vi "Launch DQMH Tools by menu.vi"(5 "Project":string="Project", 7 "Application Instance":refnum<vi>, 8 "error in":errorcluster, 10 "Module Ref":refnum<vi>, 11 "DQMH Tools":T1) -> (0 "error out":errorcluster)   [LabVIEW 2019, in "Panther Dashboard.lvlib"]
doc: "Launch a DQMH scripting tool by typing one of the following strings in Quick Drop before pressing the Ctrl-Key shortcut for this plugin:\n\nCreate New DQMH Event - ae, new event, add event, create event, \"\" (empty string)\nRename DQMH Event - re, rename event\nRemove DQMH Event - rme, remove\nConvert DQMH Event - ce, convert\nAdd New DQMH Module - am, new mod, add mod, create mod\nRename DQMH Module - rm, rename module\nValidate DQMH Module - vm, validate\nCreate DQMH Module Template - ct, template\nCreate RT Tester - crt, rt\nNew DQMH Unit Test - cut, unit\n\nDefault Shortcut - [E]"
uses:
  Panther Dashboard.lvlib
  DQMH Tools Menu--enum.ctl
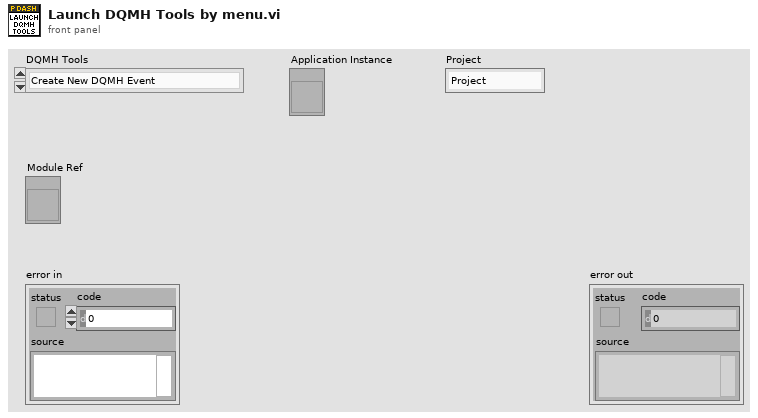
[diagram p1: front panel]
types:
  T1 = typedef "Panther Dashboard.lvlib/DQMH Tools Menu--enum.ctl" = enum16{"Create New DQMH Event", "Remove DQMH Event", "Convert DQMH Event", "Rename DQMH Event", "Add New DQMH Module", "Create RT Tester", "Rename DQMH Module", "Validate DQMH Module", "Create DQMH Module Template", "New DQMH  Unit Test"}
  T2 = enum32{"Invalid", "Standard", "Closed", "Hidden", "Minimized", "Maximized"}
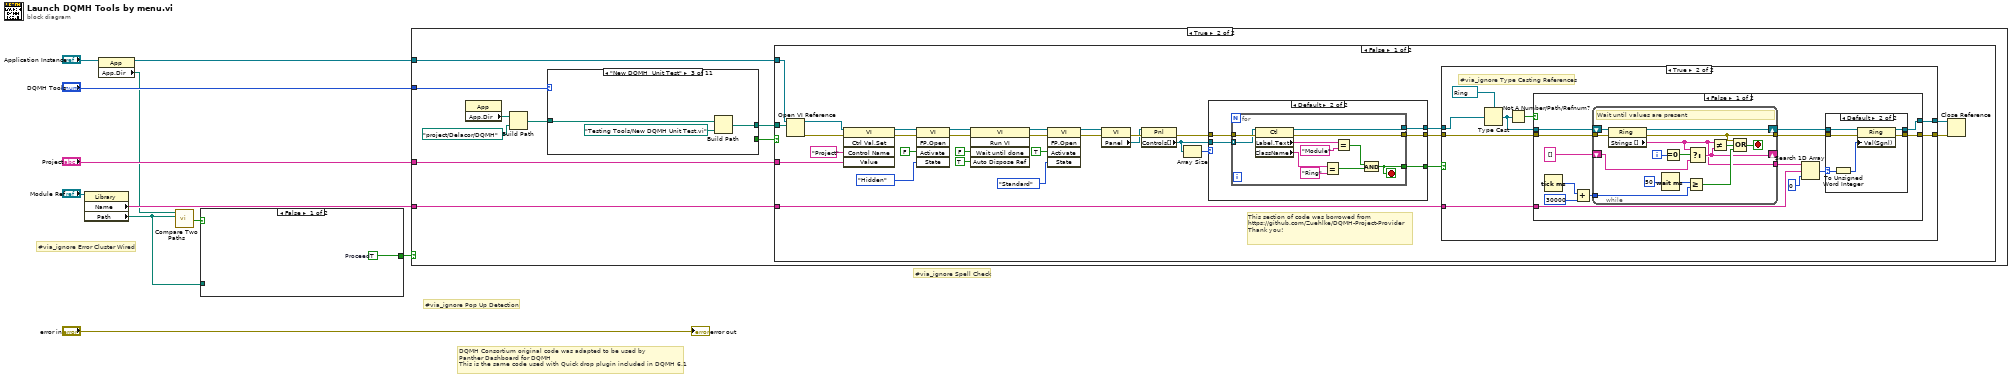
[diagram p0: block diagram]
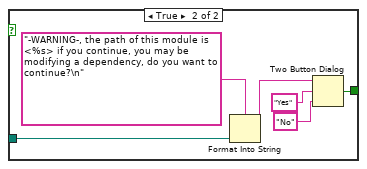
[diagram p2: hidden frame]
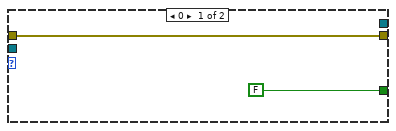
[diagram p4: hidden frame]
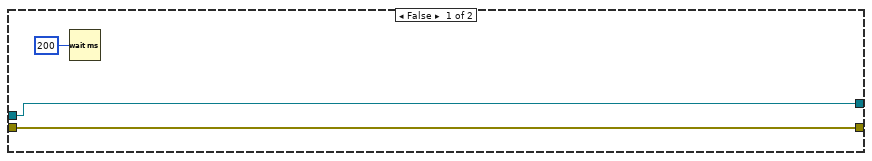
[diagram p5: hidden frame]
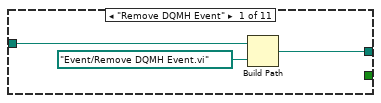
[diagram p9: hidden frame]
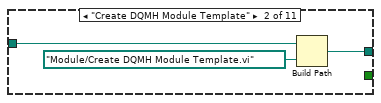
[diagram p10: hidden frame]
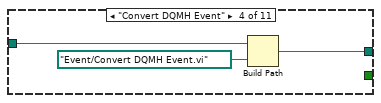
[diagram p11: hidden frame]
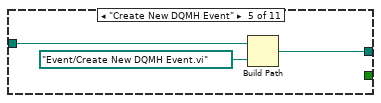
[diagram p12: hidden frame]
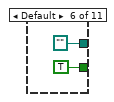
[diagram p13: hidden frame]
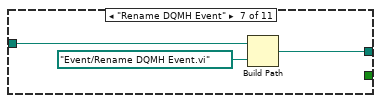
[diagram p14: hidden frame]
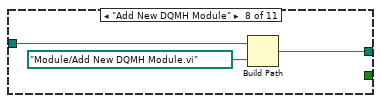
[diagram p15: hidden frame]
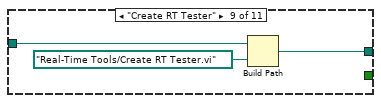
[diagram p16: hidden frame]
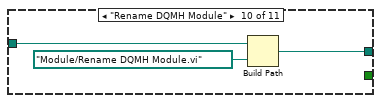
[diagram p17: hidden frame]
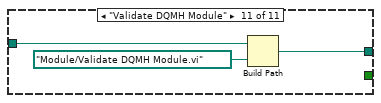
[diagram p18: hidden frame]
diagram:
  # "#via_ignore Error Cluster Wired"
  # "#via_ignore Pop Up Detection"
  # "#via_ignore Spell Check"
  # "DQMH Consortium original code was adapted to be used by \nPanther Dashboard for DQMH\nThis is the same code used with Quick drop plugin included in DQMH 6.1"
  n1 = property class="Library"(reference="Module Ref") -> ("Name"=w8:string, "Path"=w1:path)  [unwired: 1 in, 2 out]
  n2 = property class="App"(reference="Application Instance") -> (reference out=w4:refnum<vi>, "App.Dir"=w3:path)  [unwired: 1 in, 1 out]
  n3 = call <vilib>:"Compare Two Paths.vi"("Path 2"=w1, "Path 1"=w3) -> ("Path 2 Relative to Path 1?"=w2:bool)  [unwired: 6 in, 3 out]
  n4 = case shown="False" w2 {
    tunnel: [w12 w18] -> w6
    tunnel: w1 -> [_ w13]
    frame False {
      w12 = TRUE  # Proceed
    }
    frame True {
      n5 = Format Into String(format string="-WARNING-, the path of this module is <%s> if you continue, you may be modifying a dependency, do you want to continue?\n" ("message"), w13) -> (resulting string=w14:string)  [unwired: 2 in, 1 out]
      n6 = Two Button Dialog(message=w14, 1:"No" ("F button name (\"Cancel\")"), 2:"Yes" ("T button name (\"OK\")")) -> (T button?=w18:bool)
    }
  }
  n7 = case shown="True" w6 {
    tunnel: "DQMH Tools" -> [_ w23]
    tunnel: "Project" -> [_ w21]
    tunnel: w4 -> [_ w20]
    tunnel: w8 -> [_ w19]
    frame False {
    }
    frame True {
      n8 = property class="App"() -> ("App.Dir"=w27:path)  [unwired: 2 in, 2 out]
      n9 = Build Path(base path=w27, name or relative path=path "project/Delacor/DQMH" ("Application:Directory Path")) -> (appended path=w25:path)
      n10 = case shown="\"New DQMH  Unit Test\"" w23 {
        tunnel: w25 -> [w129 w132 w135 w138 w141 _ w146 w149 w152 w155 w158]
        tunnel: [w128 w131 w134 w137 w140 path "" w145 w148 w151 w154 w157] -> w24
        tunnel: [_ _ _ _ _ TRUE _ _ _ _ _] -> w22
        frame "Remove DQMH Event" {
          n11 = Build Path(base path=w129, name or relative path=path "Event/Remove DQMH Event.vi") -> (appended path=w128:path)
        }
        frame "Create DQMH Module Template" {
          n12 = Build Path(base path=w132, name or relative path=path "Module/Create DQMH Module Template.vi") -> (appended path=w131:path)
        }
        frame "New DQMH  Unit Test" {
          n13 = Build Path(base path=w135, name or relative path=path "Testing Tools/New DQMH Unit Test.vi") -> (appended path=w134:path)
        }
        frame "Convert DQMH Event" {
          n14 = Build Path(base path=w138, name or relative path=path "Event/Convert DQMH Event.vi") -> (appended path=w137:path)
        }
        frame "Create New DQMH Event" {
          n15 = Build Path(base path=w141, name or relative path=path "Event/Create New DQMH Event.vi") -> (appended path=w140:path)
        }
        frame Default {
        }
        frame "Rename DQMH Event" {
          n16 = Build Path(base path=w146, name or relative path=path "Event/Rename DQMH Event.vi") -> (appended path=w145:path)
        }
        frame "Add New DQMH Module" {
          n17 = Build Path(base path=w149, name or relative path=path "Module/Add New DQMH Module.vi") -> (appended path=w148:path)
        }
        frame "Create RT Tester" {
          n18 = Build Path(base path=w152, name or relative path=path "Real-Time Tools/Create RT Tester.vi") -> (appended path=w151:path)
        }
        frame "Rename DQMH Module" {
          n19 = Build Path(base path=w155, name or relative path=path "Module/Rename DQMH Module.vi") -> (appended path=w154:path)
        }
        frame "Validate DQMH Module" {
          n20 = Build Path(base path=w158, name or relative path=path "Module/Validate DQMH Module.vi") -> (appended path=w157:path)
        }
      }
      n21 = case shown="False" w22 {
        tunnel: w24 -> [w45 _]
        tunnel: w21 -> [w37 _]
        tunnel: w20 -> [w36 _]
        tunnel: w19 -> [w28 _]
        frame False {
          # "This section of code was borrowed from\nhttps://github.com/Zuehlke/DQMH-Project-Provider\nThank you!"
          n22 = Open VI Reference(application reference (local)=w36, vi path=w45) -> (vi reference=w49:refnum<vi>, error out=w58:errorcluster)  [unwired: 4 in]
          n23 = invoke class="VI" method="Ctrl Val.Set"(reference=w49, error in=w58, "Control Name"="Project", "Value"=w37) -> (reference out=w47:refnum<vi>, error out=w57:errorcluster)  [unwired: 1 in, 3 out]
          n24 = invoke class="VI" method="FP.Open"(reference=w47, error in=w57, "Activate"=FALSE ("Wait Until Done"), "State"=T2."Hidden") -> (reference out=w43:refnum<vi>, error out=w56:errorcluster)  [unwired: 1 in, 3 out]
          n25 = invoke class="VI" method="Run VI"(reference=w43, error in=w56, "Wait until done"=FALSE ("Wait Until Done"), "Auto Dispose Ref"=TRUE ("Auto Dispose Reference")) -> (reference out=w40:refnum<vi>, error out=w55:errorcluster)  [unwired: 1 in, 3 out]
          n26 = invoke class="VI" method="FP.Open"(reference=w40, error in=w55, "Activate"=TRUE ("Activate?"), "State"=T2."Standard") -> (reference out=w29:refnum<vi>, error out=w50:errorcluster)  [unwired: 1 in, 3 out]
          n27 = property class="VI"(reference=w29, error in=w50) -> (error out=w53:errorcluster, "Panel"=w33:refnum<vi>)  [unwired: 1 out]
          n28 = property class="Pnl"(reference=w33, error in=w53) -> (error out=w52:errorcluster, "Controls[]"=w32:refnum<vi>[])  [unwired: 1 out]
          n29 = Array Size(array=w32) -> (size(s)=w31:i32)
          n30 = case shown="Default" w31 {
            tunnel: [_ w63] -> w30
            tunnel: [FALSE w62] -> w35
            tunnel: w52 -> [w60 w65]
            tunnel: [w60 w64] -> w51
            tunnel: w32 -> [_ w61]
            frame 0 {
            }
            frame Default {
              n31 = for {
                tunnel: w61 -> [w74] mode=indexing
                tunnel: [w73] -> w63
                tunnel: [w66] -> w62
                tunnel: w65 -> [w76]
                tunnel: [w75] -> w64
                stop <- w66 stop-if-true
                n32 = property class="Ctl"(reference=w74, error in=w76) -> (reference out=w73:refnum<vi>, error out=w75:errorcluster, "Label.Text"=w72:string, "ClassName"=w70:string)
                n33 = Equal?(x=w70, y="Ring" ("Class Name")) -> (x = y?=w67:bool)
                n34 = Equal?(x=w72, y="Module" ("Control Name")) -> (x = y?=w68:bool)
                n35 = Compound Arithmetic op=AND(w68, w67) -> (w66:bool)
              }
            }
          }
          n36 = case shown="True" w35 {
            tunnel: w30 -> [w78 w85]
            tunnel: w51 -> [w79 w87]
            tunnel: [w79 w86] -> w54
            tunnel: w28 -> [_ w83]
            tunnel: [w78 w80] -> w34
            frame False {
              n37 = Wait (ms)(milliseconds to wait=u32 200) -> ()  [unwired: 1 out]
            }
            frame True {
              # "#via_ignore Type Casting References"
              n38 = Type Cast(type=refnum<vi> refnum ("Module"), x=w85) -> (*(type *) &x=w82:refnum<vi>)
              n39 = Not A Number/Path/Refnum?(number/path/refnum=w82) -> (NaN/Path/Refnum?=w81:bool)
              n40 = case shown="False" w81 {
                tunnel: w87 -> [w101 w126]
                tunnel: w83 -> [w95 _]
                tunnel: [w93 w125] -> w80
                tunnel: w82 -> [w92 w125]
                tunnel: [w99 w126] -> w86
                frame False {
                  n41 = Tick Count (ms)() -> (millisecond timer value=w89:u32)
                  n42 = Add(x=w89, y=u32 30000) -> (x+y=w88:u32)
                  n43 = while {
                    tunnel: [w103] -> w96
                    shift-right: [w114] -> w94
                    shift-left: w92 -> [w113]
                    tunnel: w101 -> [w116]
                    tunnel: [w115] -> w100
                    shift-right: [w104] -> _
                    shift-left: string[] [] ("Strings []") -> [w108]
                    tunnel: w88 -> [w102]
                    i -> [w107]
                    stop <- w111 stop-if-true
                    # "Wait until values are present"
                    n44 = property class="Ring"(reference=w113, error in=w116) -> (reference out=w114:refnum<vi>, error out=w115:errorcluster, "Strings []"=w103:string[])
                    n45 = Wait (ms)(milliseconds to wait=u32 50) -> (millisecond timer value=w110:u32)
                    n46 = Equal To 0?(x=w107) -> (x = 0?=w106:bool)
                    n47 = Greater Or Equal?(x=w110, y=w102) -> (x >= y?=w112:bool)
                    n48 = Select(t=w103, s=w106, f=w108) -> (s? t:f=w104:string[])
                    n49 = Not Equal?(x=w103, y=w104) -> (x != y?=w105:bool)
                    n50 = Compound Arithmetic op=OR(w115, w105, w112) -> (w111:bool)
                  }
                  n51 = Search 1D Array(1D array=w96, element=w95, start index (0)=0) -> (index of element=w97:i32)
                  n52 = case shown="Default" w97 {
                    selector: w97 -> [_ w122]
                    tunnel: w94 -> [w117 w121]
                    tunnel: [w117 w119] -> w93
                    tunnel: w100 -> [w118 w124]
                    tunnel: [w118 w123] -> w99
                    frame -1 {
                    }
                    frame Default {
                      n53 = To Unsigned Word Integer(number=w122) -> (unsigned 16bit integer=w120:u16)
                      n54 = property class="Ring"(reference=w121, error in=w124, "Val(Sgnl)"=w120) -> (reference out=w119:refnum<vi>, error out=w123:errorcluster)
                    }
                  }
                }
                frame True {
                }
              }
            }
          }
          n55 = Close Reference(reference=w34, error in (no error)=w54) -> ()  [unwired: 1 out]
        }
        frame True {
        }
      }
    }
  }
  "error out" <- "error in"
